vi "_get_str.vi"(3 "错误输入（无错误）":errorcluster, 4 "写入缓冲区":string, 5 "连接ID":refnum<k5>) -> (0 "错误输出":errorcluster, 1 "读取缓冲区":string, 2 "连接ID输出":refnum<k5>)   [LabVIEW 2017]
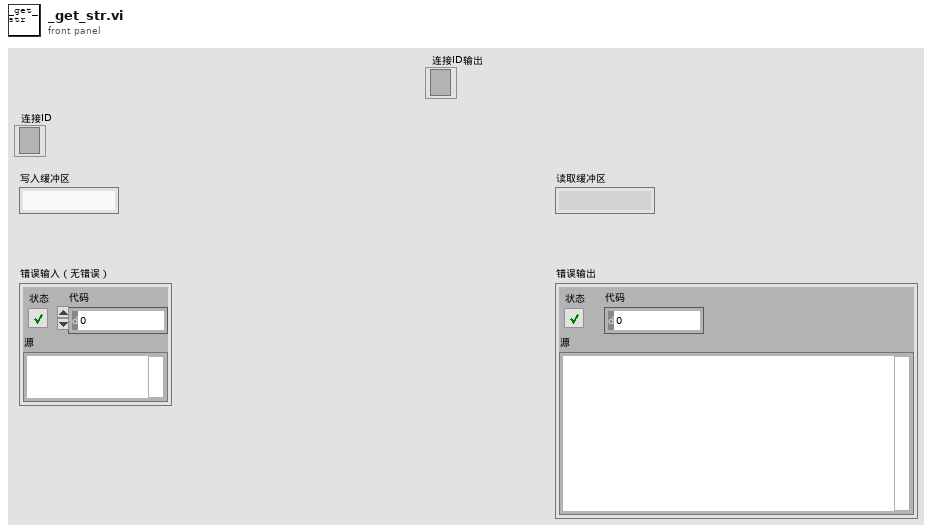
[diagram p1: front panel]
types:
  T1 = typedef "Semaphore RefNum" = refnum<k1>
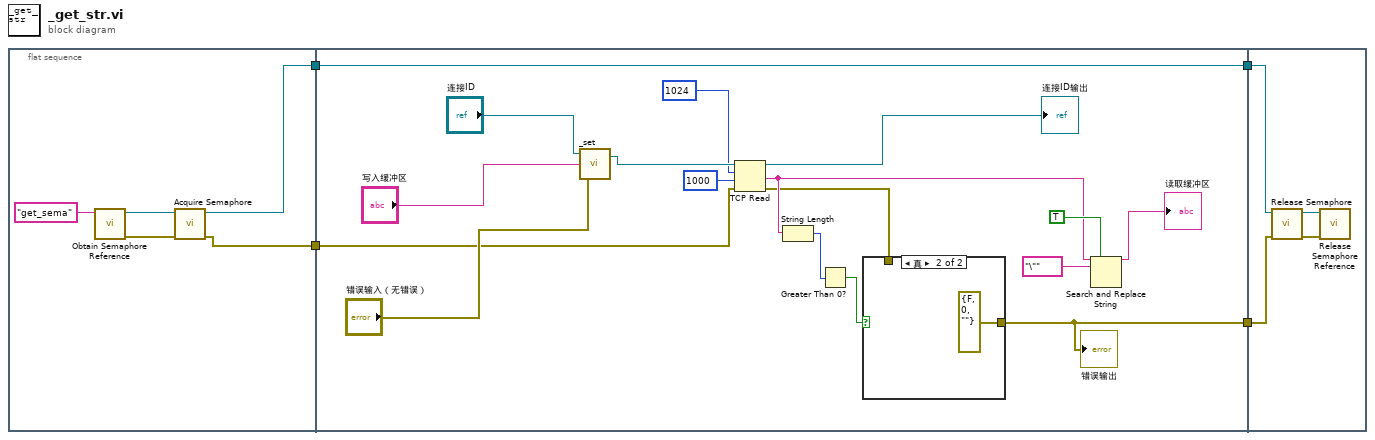
[diagram p0: block diagram]
diagram:
  n1 = flat-sequence {
    tunnel: [w7] -> w4
    tunnel: [w6] -> w3
    tunnel: w4 -> [w18]
    tunnel: w3 -> [w22]
    tunnel: [w22] -> w2
    tunnel: [w10] -> w1
    tunnel: w2 -> [w30]
    tunnel: w1 -> [w29]
    frame #0 {
      n2 = call <vilib>:"Obtain Semaphore Reference.vi"("name (unnamed)"="get_sema") -> ("error out"=w8:errorcluster, "semaphore"=w9:T1)  [unwired: 4 in, 1 out]
      n3 = call <vilib>:"Acquire Semaphore.vi"("error in (no error)"=w8, "semaphore"=w9) -> ("error out"=w7:errorcluster, "semaphore out"=w6:T1)  [unwired: 3 in, 1 out]
    }
    frame #1 {
      n4 = call "_set.vi"("错误输入（无错误）"="错误输入（无错误）", "写入缓冲区"="写入缓冲区", "连接ID"="连接ID") -> ("连接ID输出"=w20:refnum<k5>)  [unwired: 1 out]
      n5 = TCP Read(connection ID=w20, bytes to read=u32 1024 ("字节总数"), error in (no error)=w18, 9:1000 ("超时毫秒(25000)")) -> (connection ID out=→"连接ID输出":refnum<k5>, data out=w14:string, error out=w11:errorcluster)  [unwired: 1 in]
      n6 = String Length(string=w14) -> (length=w13:i32)
      n7 = Greater Than 0?(x=w13) -> (x > 0?=w12:bool)
      n8 = case shown="真" w12 {
        tunnel: [w27 errorcluster {"status"=FALSE, "code"=0, "source"=""} ("error out")] -> w10
        tunnel: w11 -> [w27 _]
        frame False {
        }
        frame True {
        }
      }
      "错误输出" <- w10
      n9 = Search and Replace String(replace all?=TRUE ("替换全部？(F)"), input string=w14, search string="\"" ("搜索字符串")) -> (result string=→"读取缓冲区":string)  [unwired: 5 in, 3 out]
    }
    frame #2 {
      n10 = call <vilib>:"Release Semaphore.vi"("error in (no error)"=w29, "semaphore"=w30) -> ("error out"=w32:errorcluster, "semaphore out"=w31:T1)  [unwired: 4 in]
      n11 = call <vilib>:"Release Semaphore Reference.vi"("error in (no error)"=w32, "semaphore"=w31) -> ()  [unwired: 8 in, 2 out]
    }
  }
